vi "OAT Probe Angle Preprocess.vi"(3 "probe angle":cluster{"X (red)":u32, "Y (blue)":u32}) -> (0 "switch x y axis":bool, 1 "probe angle out":cluster{"X (red)":dbl, "Y (blue)":dbl})   [LabVIEW 2017]
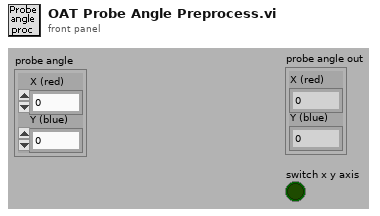
[diagram p1: front panel]
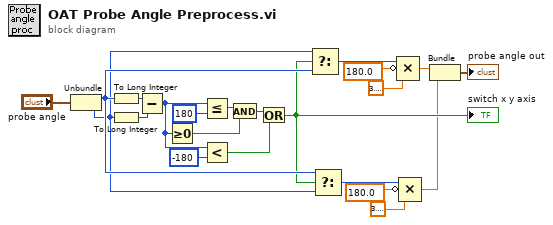
[diagram p0: block diagram]
diagram:
  n1 = Unbundle("probe angle") -> ("X (red)"=w11:u32, "Y (blue)"=w10:u32)
  n2 = To Long Integer(number=w11) -> (32bit integer=w12:i32)
  n3 = To Long Integer(number=w10) -> (32bit integer=w20:i32)
  n4 = Subtract(x=w12, y=w20) -> (x-y=w16:i32)
  n5 = Greater Or Equal To 0?(x=w16) -> (x >= 0?=w17:bool)
  n6 = Less Or Equal?(x=w16, y=u32 180) -> (x <= y?=w18:bool)
  n7 = Less?(x=w16, y=-180) -> (x < y?=w13:bool)
  n8 = And(x=w18, y=w17) -> (x .and. y?=w14:bool)
  n9 = Or(x=w14, y=w13) -> (x .or. y?=w9:bool)
  "switch x y axis" <- w9
  n10 = Select(t=w10, s=w9, f=w11) -> (s? t:f=w6:u32)
  n11 = Select(t=w11, s=w9, f=w10) -> (s? t:f=w2:u32)
  n12 = Compound Arithmetic op=MULTIPLY(w6, invert 180.0 ("value"), 3.141592653589793) -> (w5:dbl)
  n13 = Compound Arithmetic op=MULTIPLY(w2, invert 180.0 ("value"), 3.141592653589793) -> (w1:dbl)
  n14 = Bundle(w5, w1) -> (→"probe angle out":cluster{dbl, dbl})  [unwired: 1 in]
